vi "2.vi"() -> ()   [LabVIEW 2020]
panel:
  in  "STOP":bool
  out "Counter":u32
  in  "Reset(T)/Count(F)":bool
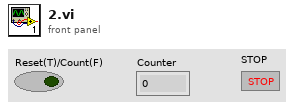
[diagram p1: front panel]
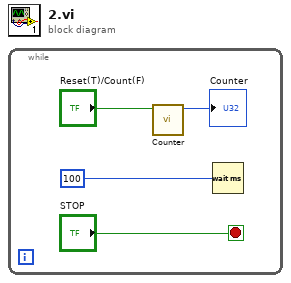
[diagram p0: block diagram]
diagram:
  n1 = while {
    stop <- "STOP" stop-if-true
    n2 = call "Counter.vi"("Reset(T)/Count(F)"="Reset(T)/Count(F)") -> ("Counter"=→"Counter":u32)  [unwired: 9 in, 1 out]
    n3 = Wait (ms)(milliseconds to wait=u32 100) -> ()  [unwired: 1 out]
  }
